vi "_QueryCommand.vi"(6 "Timeout (ms.) (3000)":u16=3000 max=10000 step=1, 7 "Disable MAV check (F)":bool, 8 "error in":errorcluster, 10 "Command":string, 11 "Instrument Channel in":string) -> (0 "error out":errorcluster, 2 "Response":string, 3 "Instrument Channel out":string)   [LabVIEW 2020, in "FCR100.lvlib"]
doc: "Query instrument with command string and read response.\n\nThis will wait for MAV bit to be set before reading over GPIB, but not with RS-232 (as this involves physically sending a command.)"
uses:
  FCR100.lvlib
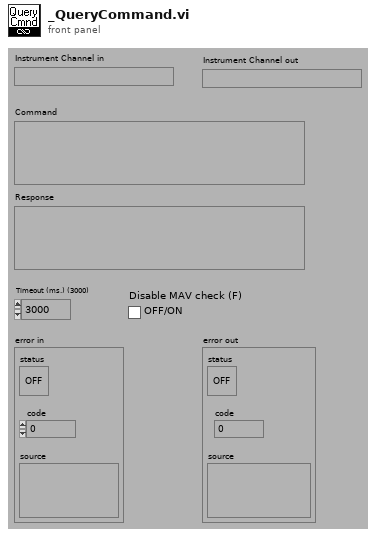
[diagram p1: front panel]
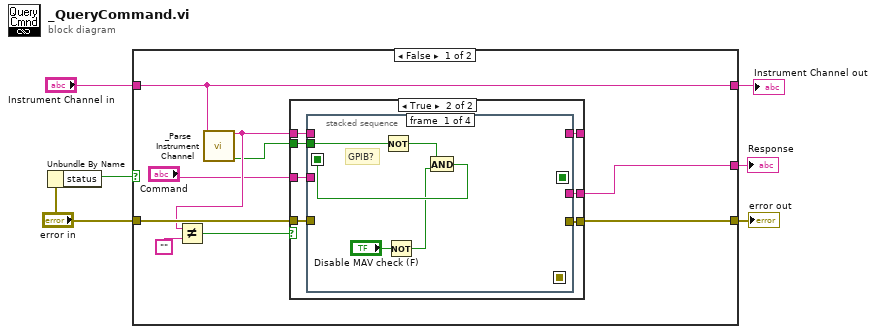
[diagram p0: block diagram]
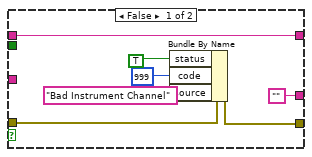
[diagram p2: hidden frame]
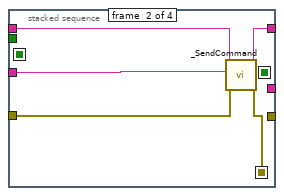
[diagram p3: hidden frame]
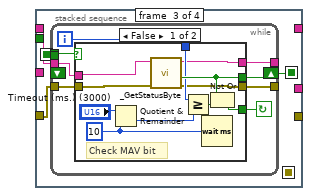
[diagram p4: hidden frame]
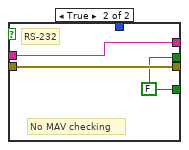
[diagram p5: hidden frame]
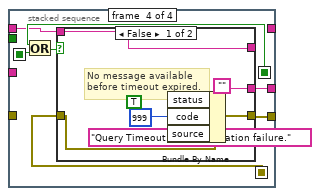
[diagram p6: hidden frame]
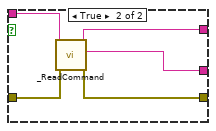
[diagram p7: hidden frame]
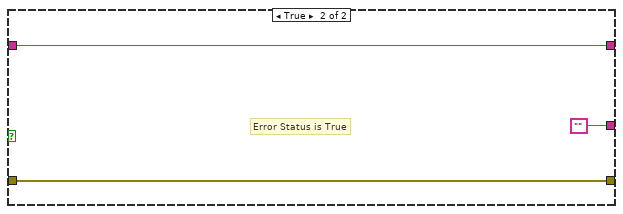
[diagram p8: hidden frame]
diagram:
  n1 = Unbundle By Name("error in") -> ("status"=w5:bool)
  n2 = case shown="False" w5 {
    tunnel: "error in" -> [w15 w86]
    tunnel: "Instrument Channel in" -> [w14 w87]
    tunnel: [w14 w87] -> w3
    tunnel: [w13 w86] -> w2
    tunnel: [w12 ""] -> w1
    frame False {
      n3 = call "_Parse Instrument Channel.vi"("Instrument Channel"=w14) -> ("T - GPIB, F - RS232"=w8:bool, "Instrument Channel out"=w9:string)  [unwired: 6 in, 3 out]
      n4 = Not Equal?(x=w9, y="") -> (x != y?=w11:bool)
      n5 = case shown="True" w11 {
        tunnel: w15 -> [w20 w28]
        tunnel: [w16 w29] -> w13
        tunnel: w9 -> [w22 w26]
        tunnel: [w22 w25] -> _
        tunnel: "Command" -> [_ w27]
        tunnel: ["" w24] -> w12
        tunnel: w8 -> [_ w23]
        frame False {
          n6 = Bundle By Name(cluster=w20, "status"=TRUE, "code"=999, "source"="Bad Instrument Channel") -> (w16:errorcluster)
        }
        frame True {
          n7 = stacked-sequence {
            seq-local: [_ _ w41 _] -> [_ _ _ w71]
            seq-local: [w34 _ _ _] -> [_ _ w40 w72]
            seq-local: [_ w36 _ _] -> [_ _ _ w67]
            tunnel: w27 -> [_ w35 _ _]
            tunnel: w28 -> [_ w39 w43 _]
            tunnel: [_ _ _ w66] -> w29
            tunnel: w26 -> [_ w38 w42 w69]
            tunnel: [_ w37 _ _] -> w25
            tunnel: [_ _ _ w68] -> w24
            tunnel: w23 -> [w31 _ _ _]
            frame #0 {
              # "GPIB?"
              n8 = Not(x=w31) -> (.not. x?=w30:bool)
              n9 = Not(x="Disable MAV check (F)") -> (.not. x?=w32:bool)
              n10 = And(x=w30, y=w32) -> (x .and. y?=w34:bool)
            }
            frame #1 {
              n11 = call "_SendCommand.vi"("error in"=w39, "Command"=w35, "Instrument Channel"=w38) -> ("error out"=w36:errorcluster, "Instrument Channel out"=w37:string)  [unwired: 7 in]
            }
            frame #2 {
              n12 = while {
                tunnel: w40 -> [w44]
                tunnel: w40 -> [_]
                shift-left: _ -> [_]
                shift-right: [w45] -> w41
                tunnel: w42 -> [w48]
                tunnel: [w49] -> _
                tunnel: [w50] -> _
                tunnel: w43 -> [w51]
                i -> [w47]
                stop <- w46 continue-if-true
                n13 = case shown="False" w44 {
                  tunnel: [w58 w63] -> w45
                  tunnel: [w57 w63] -> w46
                  tunnel: w47 -> [w56 _]
                  tunnel: w48 -> [w55 w65]
                  tunnel: [w54 w65] -> w49
                  tunnel: [w53 w64] -> w50
                  tunnel: w51 -> [w52 w64]
                  frame False {
                    w60 = 10
                    # "Check MAV bit"
                    n14 = Quotient & Remainder(x="Timeout (ms.) (3000)", y=w60) -> (floor(x/y)=w62:i32)  [unwired: 1 out]
                    n15 = call "_GetStatusByte.vi"("error in"=w52, "Instrument Channel"=w55) -> ("error out"=w53:errorcluster, "MAV bit"=w58:bool, "Instrument Channel out"=w54:string)  [unwired: 6 in, 1 out]
                    n16 = Greater Or Equal?(x=w56, y=w62) -> (x >= y?=w59:bool)
                    n17 = Wait (ms)(milliseconds to wait=w60) -> ()  [unwired: 1 out]
                    n18 = Not Or(1:w59, 2:w58) -> (0:w57:bool)
                  }
                  frame True {
                    w63 = FALSE
                    # "No MAV checking"
                    # "RS-232"
                  }
                }
              }
            }
            frame #3 {
              n19 = Or(x=w71, y=w72) -> (x .or. y?=w70:bool)
              n20 = case shown="False" w70 {
                tunnel: w67 -> [w73 w84]
                tunnel: [w74 w83] -> w66
                tunnel: [w79 w82] -> _
                tunnel: w69 -> [w79 w81]
                tunnel: ["" w80] -> w68
                frame False {
                  # "No message available\nbefore timeout expired."
                  n21 = Bundle By Name(cluster=w73, "status"=TRUE, "code"=999, "source"="Query Timeout - Communication failure.") -> (w74:errorcluster)
                }
                frame True {
                  n22 = call "_ReadCommand.vi"("error in"=w84, "Instrument Channel"=w81) -> ("error out"=w83:errorcluster, "Response"=w80:string, "Instrument Channel out"=w82:string)  [unwired: 7 in]
                }
              }
            }
          }
        }
      }
    }
    frame True {
      # "Error Status is True"
    }
  }
  "Instrument Channel out" <- w3
  "error out" <- w2
  "Response" <- w1
